vi "UDP - Reciever - 2 D array.vi"() -> ()   [LabVIEW 2016]
doc: "The UDP protocol differs from TCP in that there is no error-checking with the packets of information that are sent, and thus no guarantee whatsoever that an intended recipient will actually receive a given piece of data.\n\nUDP does offer the ability to \"broadcast\" data across a network--simply specify an IP Address of all ones (255.255.255.255) to attempt to broadcast information network-wide. Keep in mind that routers and other network hardware will generally refuse to forward the broadcast beyond certain points, so the extent of the broadcast will in practice be limited."
panel:
  out "size(s)":i32[](array[numeric])
  out "value":dbl[][](array[numeric])
  in  "Stop":bool
  # "Overview: Demonstrates the use of the UDP functions to receive data over a UDP connection.\nInstructions:\n1. Ensure Simple UDP - Sender.vi is already running.\n2. Run the VI.\n3. Click Stop to stop the VI."
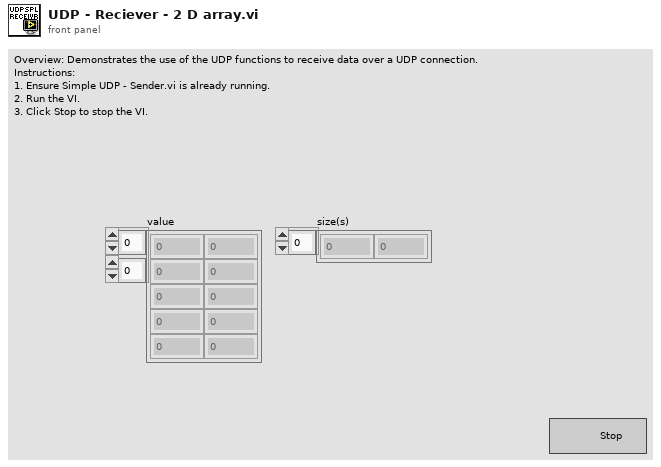
[diagram p1: front panel]
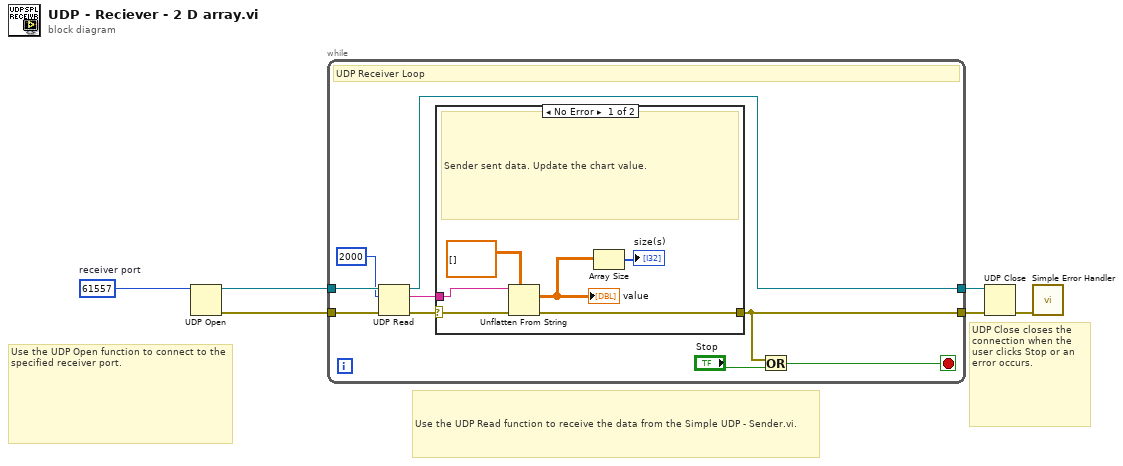
[diagram p0: block diagram]
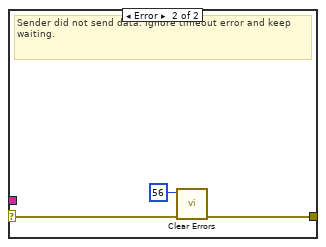
[diagram p2: hidden frame]
diagram:
  w1 = u16 61557  # receiver port
  # "UDP Close closes the connection when the user clicks Stop or an error occurs."
  # "Use the UDP Open function to connect to the specified receiver port."
  # "Use the UDP Read function to receive the data from the Simple UDP - Sender.vi."
  n1 = UDP Open(11:w1) -> (port=w2:refnum<k16>, 0:w3:errorcluster)  [unwired: 4 in, 1 out]
  n2 = while {
    tunnel: w2 -> [w15]
    tunnel: [w8] -> w6
    tunnel: w3 -> [w12]
    tunnel: [w9] -> w4
    stop <- w13 stop-if-true
    # "UDP Receiver Loop"
    n3 = UDP Read(connection ID=w15, max size (548)=2000, 8:w12) -> (data out=w11:string, error out=w10:errorcluster, 3:w8:refnum<k16>)  [unwired: 1 in, 2 out]
    n4 = case shown="No Error" w10 {
      selector: w10 -> [w21 w24]
      tunnel: w11 -> [w20 _]
      tunnel: [w16 w23] -> w9
      frame No Error {
        # "Sender sent data. Update the chart value."
        n5 = Unflatten From String(type=dbl[][] [], binary string=w20, error in (no error)=w21) -> (value=w18:dbl[][], error out=w16:errorcluster)  [unwired: 2 in, 1 out]
        "value" <- w18
        n6 = Array Size(array=w18) -> (size(s)=→"size(s)":i32[])
      }
      frame Error {
        # "Sender did not send data. Ignore timeout error and keep waiting."
        n7 = call <vilib>:"Clear Errors.vi"("error in (no error)"=w24, "specific error code to clear (0: all)"=56) -> ("error out"=w23:errorcluster)  [unwired: 4 in, 1 out]
      }
    }
    n8 = Or(x=w9, y="Stop") -> (x .or. y?=w13:bool)
  }
  n9 = UDP Close(connection ID=w6, 8:w4) -> (error out=w5:errorcluster)  [unwired: 1 out]
  n10 = call <vilib>:"Simple Error Handler.vi"("error in (no error)"=w5) -> ()  [unwired: 1 in, 8 out]
